vi "To Variant.vi"(0 "Obj in":refnum<class "Waveform.lvclass">, 11 "error in (no error)":errorcluster) -> (4 "Obj out":refnum<class "Waveform.lvclass">, 8 "Array":variant[](array[variant]), 15 "error out":errorcluster)   [LabVIEW 2020, in "Waveform.lvclass"]
uses:
  Waveform.lvclass
  D:/Development/epl-vi-lib/Koop/KObject Class/KObject.lvclass
  Waveform.lvclass/Waveform.ctl
  Koop/KObject Class/KObject.lvclass
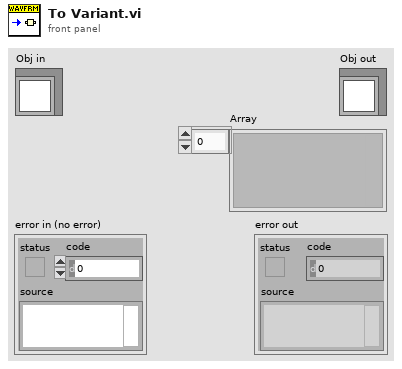
[diagram p1: front panel]
types:
  T1 = typedef "Waveform.lvclass/Serialized.ctl" = cluster{"Numeric":dbl}
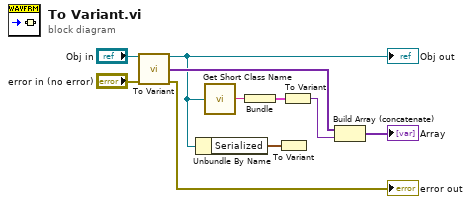
[diagram p0: block diagram]
diagram:
  n1 = call-parent "To Variant.vi"("KObject in"="Obj in", "error in (no error)"="error in (no error)") -> ("KObject out"=w4:refnum<class "Waveform.lvclass">, "Array"=w6:variant[], "error out"=→"error out":errorcluster)  [unwired: 11 in]
  "Obj out" <- w4
  n2 = Unbundle By Name(w4) -> ("Serialized"=w7:T1)
  n3 = call "Get Short Class Name.vi"("KObject in"=w4) -> ("Class"=w3:string)  [unwired: 4 in]
  n4 = Bundle("Class"=w3) -> (w2:cluster{"Class":string})  [unwired: 1 in]
  n5 = To Variant(anything=w7) -> ()  [unwired: 1 out]
  n6 = To Variant(anything=w2) -> (Variant=w1:variant)
  n7 = Build Array (concatenate)(w6, w1) -> (→"Array":variant[])
